vi "Create Measurement.vi"(8 "error in":errorcluster) -> (0 "error out":errorcluster, 3 "gRPCid out":T1)   [LabVIEW 2025, in "Automotive Ethernet Bus Monitor_LabVIEW.lvlib"]
doc: "Create client for the measurement service and complete metadata registration."
uses:
  Automotive Ethernet Bus Monitor_LabVIEW.lvlib
  <vilib>/gRPC/LabVIEW gRPC Library/Shared/grpcId.ctl
  <vilib>/gRPC/Generated APIs/ni/measurementlink/discovery/v1/RPC Messages/ni_measurementlink_discovery_v1_ResolveServiceRequest.ctl
  controls/Measurement Results.ctl
  controls/Measurement Configuration.ctl
  <vilib>/Plug-In SDKs/Clients/Discovery V1/NI Discovery V1 Client.lvlib
  <vilib>/gRPC/Generated APIs/ni/measurementlink/discovery/v1/ni.measurementlink.discovery.v1.api.lvlib
  <vilib>/gRPC/LabVIEW gRPC Library/grpc-lvsupport-release.lvlib
  <vilib>/gRPC/Generated APIs/ni/measurementlink/measurement/v2/Measurement Service Client V2/Measurement Service Client V2.lvlib
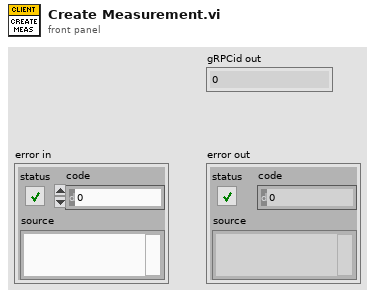
[diagram p1: front panel]
types:
  T1 = typedef "grpc-lvsupport-release.lvlib/grpcId.ctl" = u64
  T2 = typedef "Automotive Ethernet Bus Monitor_LabVIEW.lvlib/Measurement Configuration.ctl" = cluster{"double array in":dbl[], "double in":dbl, "U32 array in":u32[], "U32 in":u32, "U64 array in":u64[], "U64 in":u64, "I32 array in":i32[], "I32 in":i32, "I64 array in":i64[], "I64 in":i64, "bool in":bool, "string in":string, "u32 color ring in":u32, "u32 animal enum in":enum32{"Rabbit", "Gopher", "Badger"}}
  T3 = typedef "Automotive Ethernet Bus Monitor_LabVIEW.lvlib/Measurement Results.ctl" = cluster{"xy data out":cluster{"x_data":dbl[], "y_data":dbl[]}, "double array out":dbl[], "double out":dbl, "U32 array out":u32[], "U32 out":u32, "U64 array out":u64[], "U64 out":u64, "I32 array out":i32[], "I32 out":i32, "I64 array out":i64[], "I64 out":i64, "bool out":bool, "string out":string, "u32 color ring out":u32, "u32 animal enum out":enum32{"Rabbit", "Gopher", "Badger"}}
  T4 = typedef "ni.measurementlink.discovery.v1.api.lvlib/ni_measurementlink_discovery_v1_ResolveServiceRequest.ctl" = cluster{"provided_interface":string, "service_class":string, "deployment_target":string, "version":string}
  T5 = typedef "ni.measurementlink.discovery.v1.api.lvlib/ni_measurementlink_discovery_v1_ServiceLocation.ctl" = cluster{"location":string, "insecure_port":string, "ssl_authenticated_port":string}
  T6 = typedef "grpc-lvsupport-release.lvlib/Enum Metadata.ctl" = cluster{"Version":i32, "Name":string, "Type Url":string, "Enum Values":string, "Allow Alias":bool}
  T7 = typedef "grpc-lvsupport-release.lvlib/Message Metadata.ctl" = cluster{"Version":i32, "Name":string, "Type Url":string, "Elements":T8[], "Has Oneof":bool}
  T8 = typedef "grpc-lvsupport-release.lvlib/Message Element Metadata.ctl" = cluster{"Field Name":string, "Embedded Message Name":string, "Protobuf Index":i32, "MessageElementType":T9, "Repeated":bool, "Is in Oneof":bool, "Oneof Container Name":string}
  T9 = typedef "grpc-lvsupport-release.lvlib/Message Element Type.ctl" = enum32{"Int32Value", "FloatValue", "DoubleValue", "BoolValue", "StringValue", "MessageValue", "Int64Value", "UInt32Value", "UInt64Value", "EnumValue", "Bytes", "Fixed64", "Fixed32", "SFixed64", "SFixed32", "SInt64", "SInt32"}
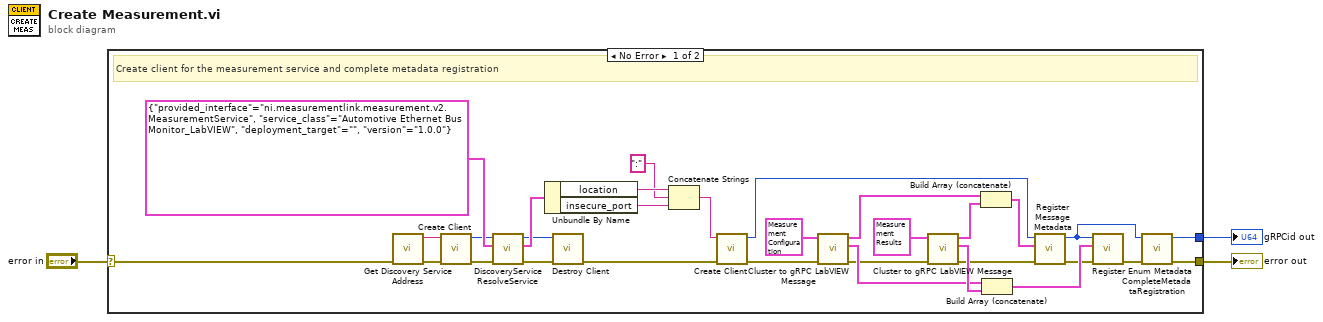
[diagram p0: block diagram]
diagram:
  n1 = case shown="No Error" "error in" {
    selector: "error in" -> [w31 w35]
    tunnel: [w15 w35] -> w2
    tunnel: [w14 _] -> w1
    frame No Error {
      # "Create client for the measurement service and complete metadata registration"
      n2 = call <vilib>:"Get Discovery Service Address.vi"("error in"=w31) -> ("error out"=w32:errorcluster, "address"=w33:string)  [unwired: 9 in]
      n3 = call <vilib>:"Create Client.vi"("error in"=w32, "address"=w33) -> ("error out"=w30:errorcluster, "gRPC ID Out"=w6:T1)  [unwired: 8 in]
      n4 = call <vilib>:"DiscoveryService ResolveService.vi"("error in"=w30, "Request Data"=T4 {"provided_interface"="ni.measurementlink.measurement.v2.MeasurementService", "service_class"="Automotive Ethernet Bus Monitor_LabVIEW", "deployment_target"="", "version"="1.0.0"} ("resolve service request data"), "gRPC ID"=w6) -> ("error out"=w27:errorcluster, "Response Data"=w29:T5, "gRPC ID out"=w28:T1)  [unwired: 6 in]
      n5 = Unbundle By Name(w29) -> ("location"=w11:string, "insecure_port"=w10:string)
      n6 = call <vilib>:"Destroy Client.vi"("error in"=w27, "gRPC ID"=w28) -> ("error out"=w26:errorcluster)  [unwired: 9 in]
      n7 = Concatenate Strings(w11, ":" ("string"), w10) -> (w9:string)
      n8 = call <vilib>:"Create Client.vi"("error in"=w26, "address"=w9) -> ("error out"=w13:errorcluster, "gRPC ID Out"=w20:T1)  [unwired: 8 in]
      n9 = call <vilib>:"Cluster to gRPC LabVIEW Message.vi"("error in"=w13, "Cluster"=T2 {"double array in"=[], "double in"=0.0, "U32 array in"=[], "U32 in"=0, "U64 array in"=[], "U64 in"=0, "I32 array in"=[], "I32 in"=0, "I64 array in"=[], "I64 in"=0, "bool in"=FALSE, "string in"="", "u32 color ring in"=0, "u32 animal enum in"=enum."Rabbit"} ("ConfigurationParameter")) -> ("error out"=w12:errorcluster, "gRPC Enum Metadata out"=w24:T6[], "gRPC Message Metadata []"=w19:T7[])  [unwired: 7 in]
      n10 = call <vilib>:"Cluster to gRPC LabVIEW Message.vi"("error in"=w12, "Cluster"=T3 {"xy data out"={"x_data"=[], "y_data"=[]}, "double array out"=[], "double out"=0.0, "U32 array out"=[], "U32 out"=0, "U64 array out"=[], "U64 out"=0, "I32 array out"=[], "I32 out"=0, "I64 array out"=[], "I64 out"=0, "bool out"=FALSE, "string out"="", "u32 color ring out"=0, "u32 animal enum out"=enum."Rabbit"} ("OutputParameter")) -> ("error out"=w16:errorcluster, "gRPC Enum Metadata out"=w25:T6[], "gRPC Message Metadata []"=w17:T7[])  [unwired: 7 in]
      n11 = Build Array (concatenate)(w19, w17) -> (w18:T7[])
      n12 = Build Array (concatenate)(w24, w25) -> (w23:T6[])
      n13 = call <vilib>:"Register Message Metadata.vi"("error in"=w16, "Messages"=w18, "gRPCid in"=w20) -> ("error out"=w21:errorcluster, "gRPCid out"=w34:T1)  [unwired: 7 in]
      n14 = call <vilib>:"Register Enum Metadata.vi"("error in"=w21, "Enum Metadata"=w23, "gRPCid in"=w34) -> ("error out"=w22:errorcluster)  [unwired: 7 in, 1 out]
      n15 = call <vilib>:"CompleteMetadataRegistration.vi"("error in"=w22, "gRPC ID in"=w34) -> ("error out"=w15:errorcluster, "gRPC ID Out"=w14:T1)  [unwired: 8 in]
    }
    frame Error {
      # "Pass"
    }
  }
  "error out" <- w2
  "gRPCid out" <- w1
